vi "Read Time Stamp.vi"(8 "error in (no error)":errorcluster, 11 "Data Message in":refnum<class "Data Message.lvclass">) -> (0 "error out":errorcluster, 2 "Time Stamp":timestamp, 3 "Data Message out":refnum<class "Data Message.lvclass">)   [LabVIEW 2020, in "Wrapped Actor.lvlib" / "Data Message.lvclass"]
uses:
  Data Message.lvclass
  Data Message.lvclass/Data Message.ctl
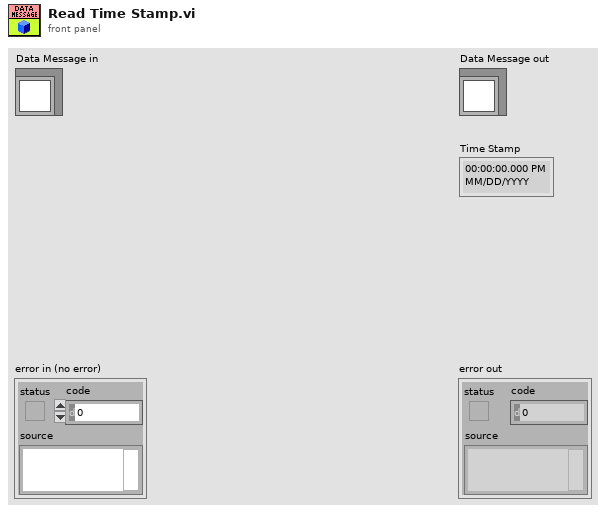
[diagram p1: front panel]
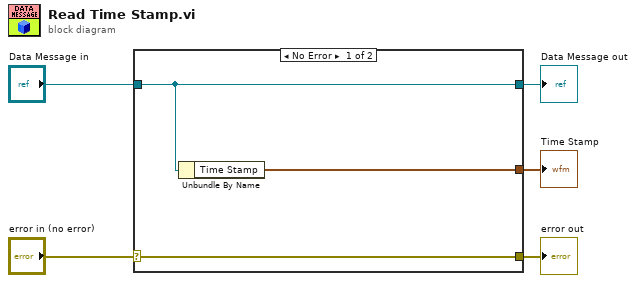
[diagram p0: block diagram]
diagram:
  n1 = case shown="No Error" "error in (no error)" {
    selector: "error in (no error)" -> [w8 w9]
    tunnel: [w8 w9] -> w4
    tunnel: [w7 w10] -> w2
    tunnel: "Data Message in" -> [w7 w10]
    tunnel: [w6 _] -> w1
    frame No Error {
      n2 = Unbundle By Name(w7) -> ("Time Stamp"=w6:timestamp)
    }
    frame Error {
    }
  }
  "error out" <- w4
  "Data Message out" <- w2
  "Time Stamp" <- w1
